vi "ObtainQueue.vi"(8 "Error In":errorcluster[](array[cluster]), 10 "BC ID":i32) -> (0 "Error Out":errorcluster[](array[cluster]), 3 "QueRef":refnum<queue>)   [LabVIEW 2017, in "BusController.lvlib"]
uses:
  BusController.lvlib
  QueueType.ctl
  <userlib>/NIST/NISTErrorLib/NISTErrorLib.lvlib
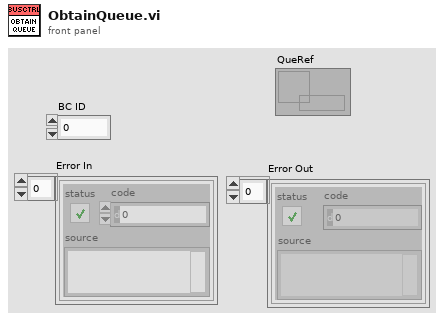
[diagram p1: front panel]
types:
  T1 = typedef "BusController.lvlib/QueueType.ctl" = cluster{"Msg":string, "Data":variant}
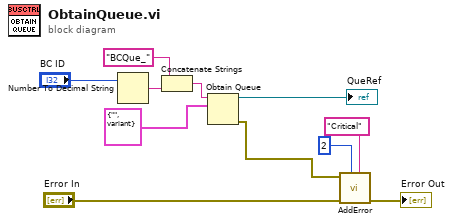
[diagram p0: block diagram]
diagram:
  n1 = Number To Decimal String(number="BC ID") -> (decimal integer string=w3:string)  [unwired: 1 in]
  n2 = Concatenate Strings("BCQue_" ("name (unnamed)"), w3) -> (w2:string)
  n3 = Obtain Queue(name (unnamed)=w2, element data type=T1 {"Msg"="", "Data"=variant} ("QueueType")) -> (queue out=→"QueRef":refnum<queue>, error out=w5:errorcluster)  [unwired: 3 in, 1 out]
  n4 = call <userlib>:"AddError.vi"("Severity"="Critical", "Priority"=u8 2, "ErrorArray"="Error In", "error in (no error)"=w5) -> ("ErrorArray"=→"Error Out":errorcluster[])  [unwired: 6 in, 1 out]
